vi "set dhe parameters.vi"(8 "error in":errorcluster, 10 "parameters":string, 11 "lvlibretls configurable context in":refnum<class "lvlibretls configurable context.lvclass">) -> (0 "error out":errorcluster, 3 "lvlibretls configurable context out":refnum<class "lvlibretls configurable context.lvclass">)   [LabVIEW 2016, in "lvlibretls configurable context.lvclass"]
uses:
  lvlibretls configurable context.lvclass
  lvlibretls configurable context.lvclass/lvlibretls configurable context.ctl
  lv tls dll.lvlib
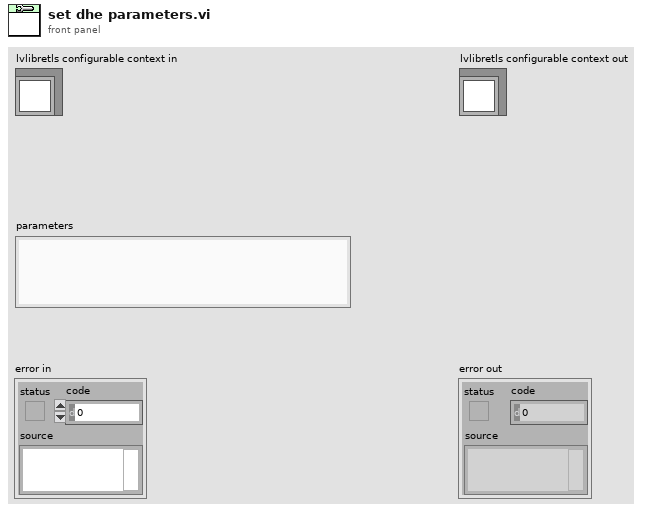
[diagram p1: front panel]
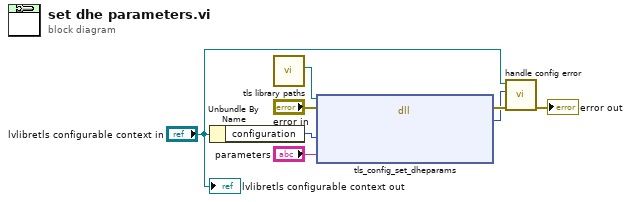
[diagram p0: block diagram]
diagram:
  n1 = Unbundle By Name("lvlibretls configurable context in") -> ("configuration"=w7:u64)
  n2 = call "tls library paths.vi"() -> ("libtls"=w8:path)  [unwired: 8 in, 3 out]
  n3 = dll-call lib="C:/Users/IEUser/Desktop/tlssimple/libtls-15.dll" fn="tls_config_set_dheparams"(path in=w8, error in="error in", "config"=w7, "parameters"="parameters") -> (error out=w6:errorcluster, "return"=w5:i32)  [unwired: 3 in, 1 out]
  n4 = call "handle config error.vi"("error in"=w6, "return"=w5, "lvlibretls configurable context in"="lvlibretls configurable context in") -> ("error out"=→"error out":errorcluster)  [unwired: 8 in]
  "lvlibretls configurable context out" <- "lvlibretls configurable context in"
